vi "MicronManager.vi"() -> ()   [LabVIEW 2019]
uses:
  MicronManager.lvclass
  <vilib>/Utility/error.llb/DialogType.ctl
  <vilib>/SLL Toolkit/SLL Queued State Machine/Queue Driver/Create Queue.vi
  <vilib>/SLL Toolkit/SLL Queued State Machine/Queue Driver/Enqueue an Item to Queue.vi
  <vilib>/SLL Toolkit/SLL Queued State Machine/Queue Driver/Dequeue Queue.vi
  <vilib>/SLL Toolkit/SLL Queued State Machine/Queue Driver/Enqueue N Items.vi
  <vilib>/SLL Toolkit/SLL Easy TCP/_SubVIs/TCP Initialize Client - Local.vi
  <vilib>/SLL Toolkit/SLL String/_SubVIs/I32 to String.vi
  <vilib>/SLL Toolkit/SLL Queued State Machine/Queue Driver/Flush Queue.vi
  <vilib>/SLL Toolkit/SLL Queued State Machine/Queue Driver/Release Queue.vi
  <vilib>/SLL Toolkit/SLL Easy TCP/SLL Easy API via TCP.lvclass
  <vilib>/SLL Toolkit/SLL Queued State Machine/SLL QSM.lvlib
  <vilib>/SLL Toolkit/SLL String/SLL String.lvlib
panel:
  in  "Ping All":bool
  out "Status":string
  in  "Tab Control":enum32{"Services", "Message"}(tab)
  out "Services":string[][](table)
  in  "Service Name":string(combo)="MicronService"
  out "Read Data":string
  in  "Command":string(combo)="Ping"
  in  "Execute":bool
  in  "Service List":path=path "ServiceList.csv"
  in  "Stop All":bool
  in  "Start All":bool
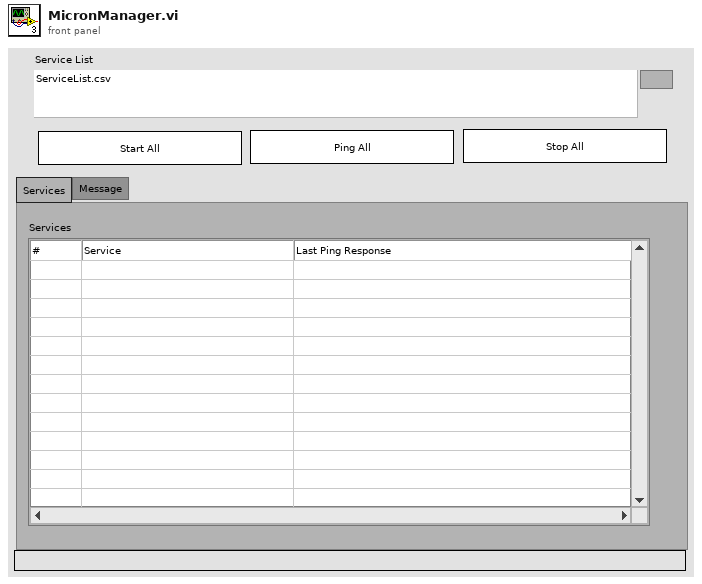
[diagram p1: front panel]
types:
  T1 = cluster{"Flags":cluster{"Source Code?":bool}, "Services":string[], "MicronManager":refnum<class "MicronManager.lvclass">, "Ping Responses":string[]}
  T2 = typedef "DialogType.ctl" = u16
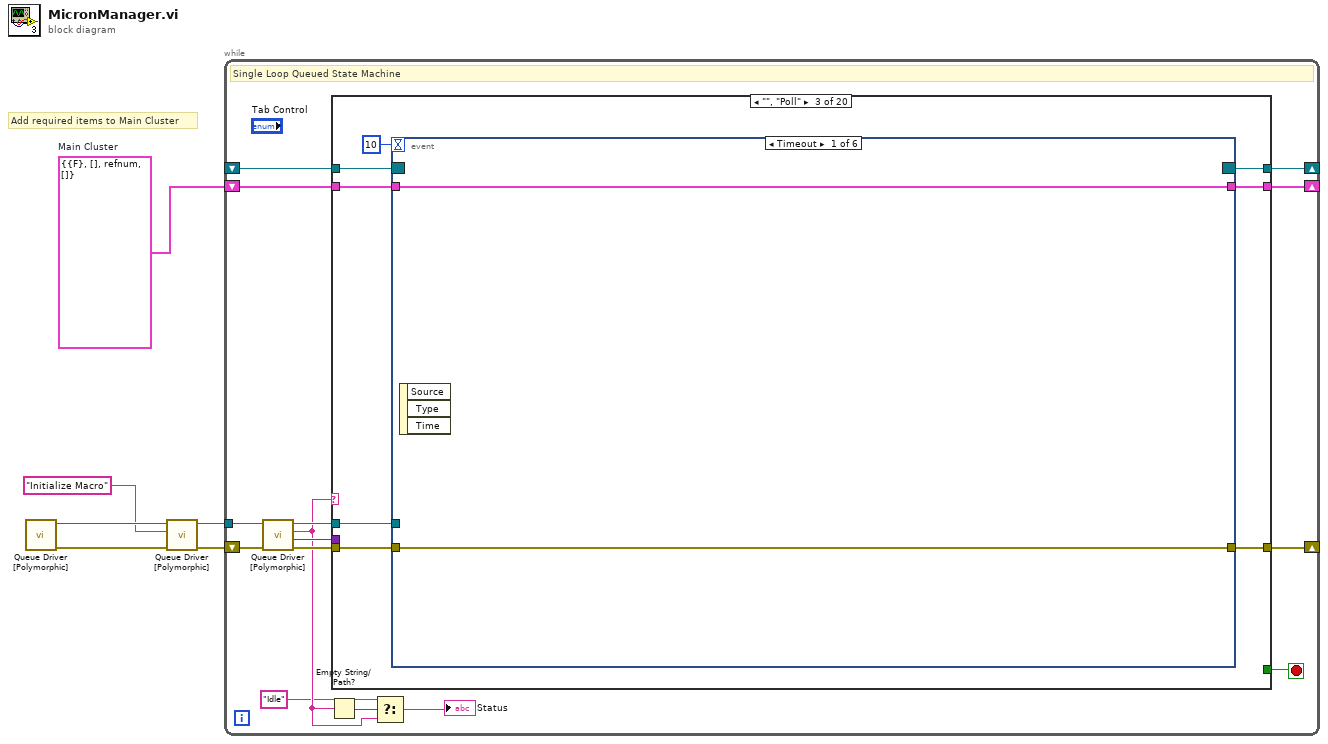
[diagram p0: block diagram]
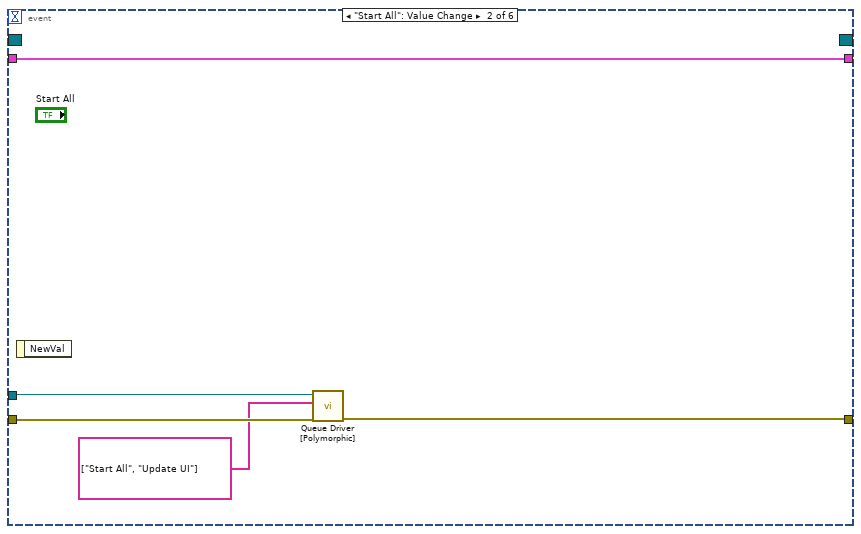
[diagram p4: hidden frame]
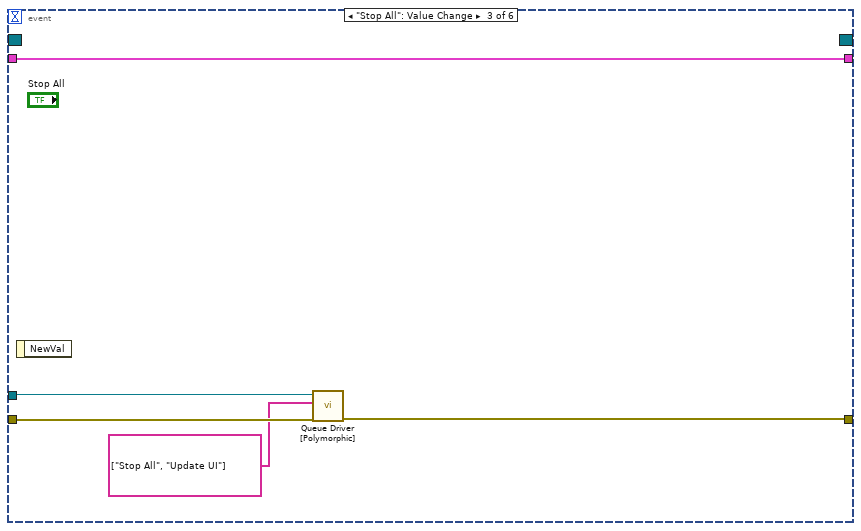
[diagram p5: hidden frame]
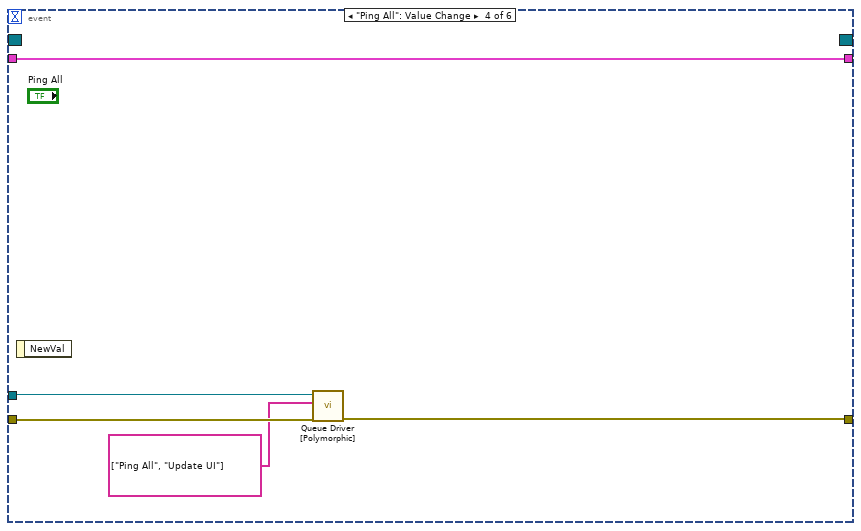
[diagram p6: hidden frame]
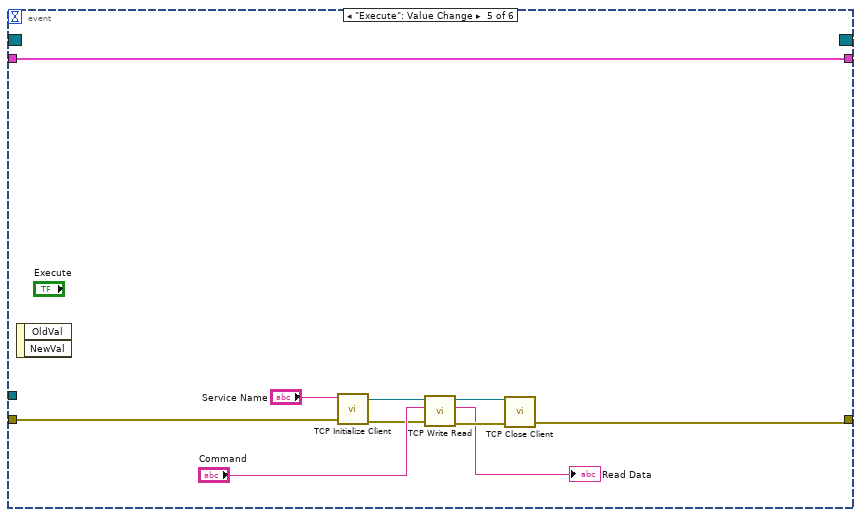
[diagram p7: hidden frame]
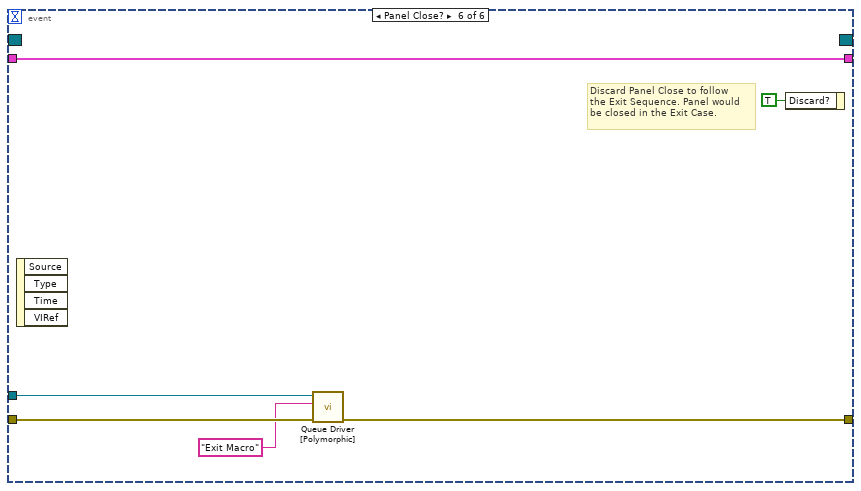
[diagram p8: hidden frame]
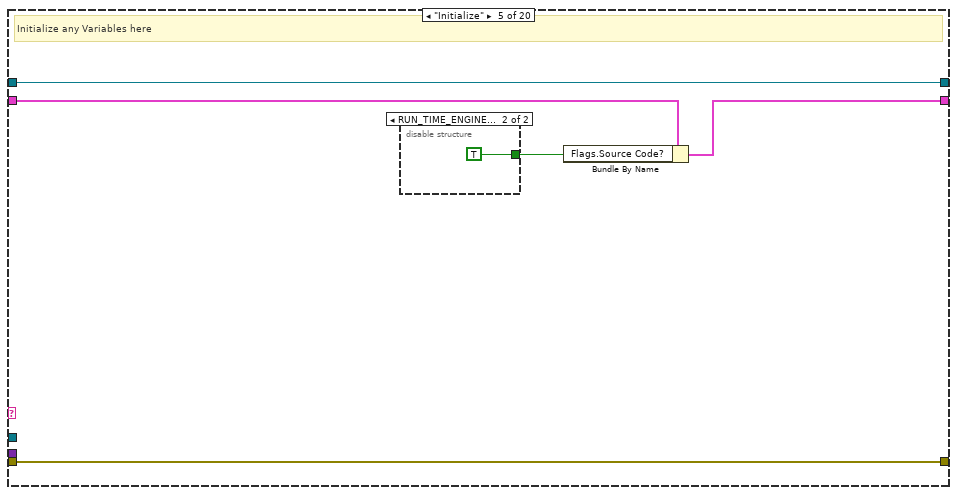
[diagram p10: hidden frame]
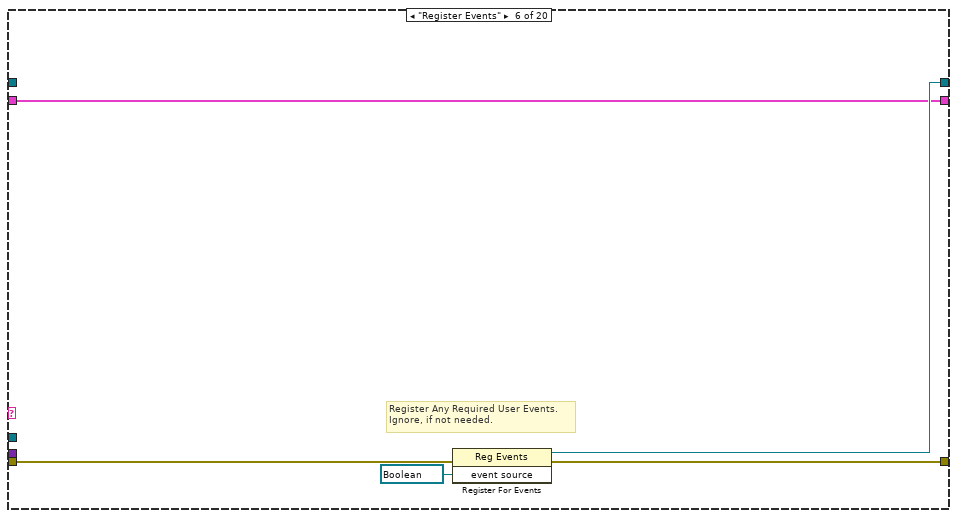
[diagram p12: hidden frame]
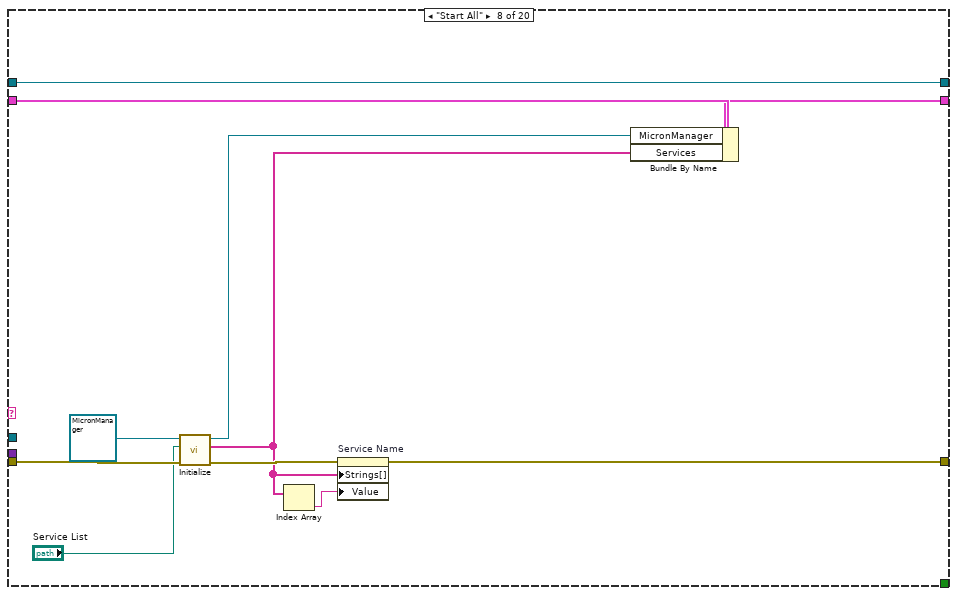
[diagram p14: hidden frame]
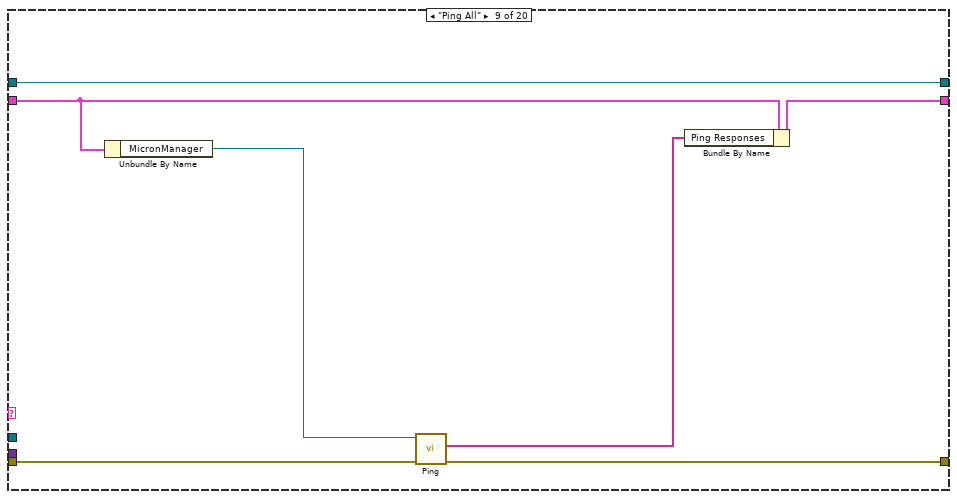
[diagram p15: hidden frame]
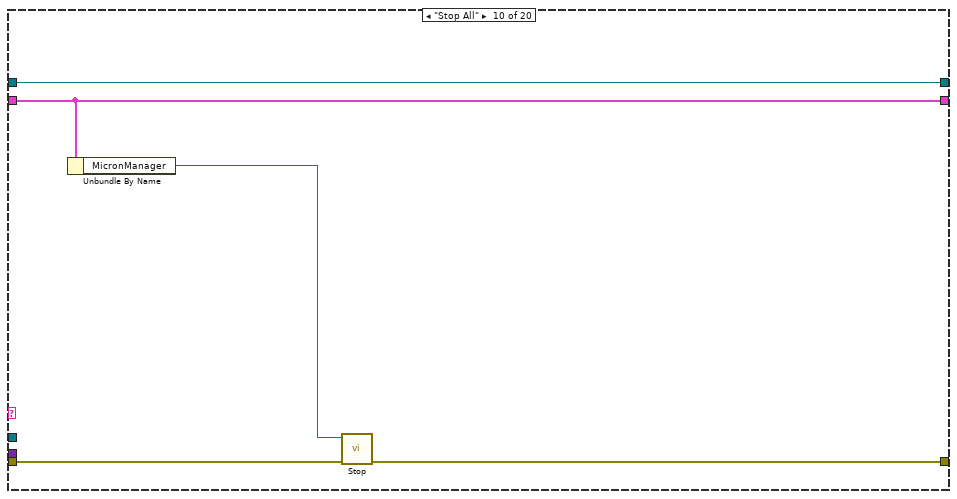
[diagram p16: hidden frame]
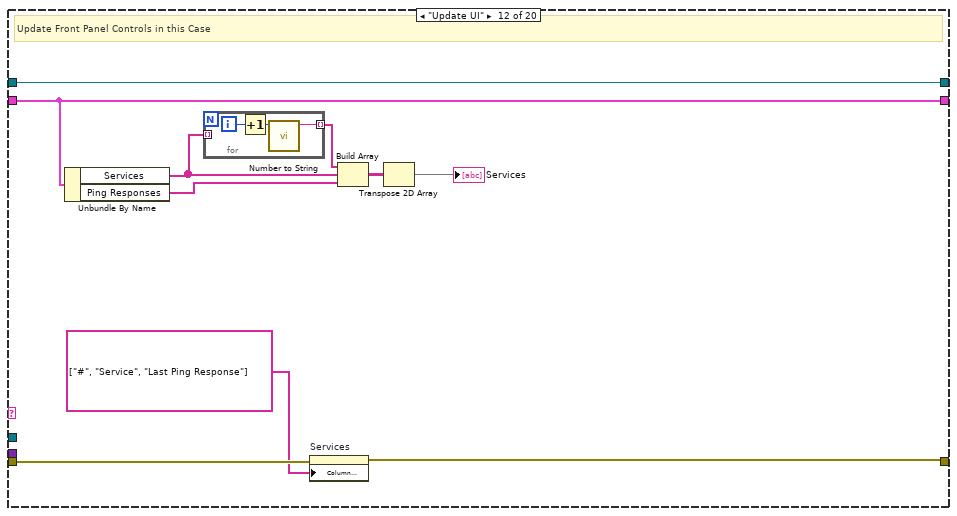
[diagram p18: hidden frame]
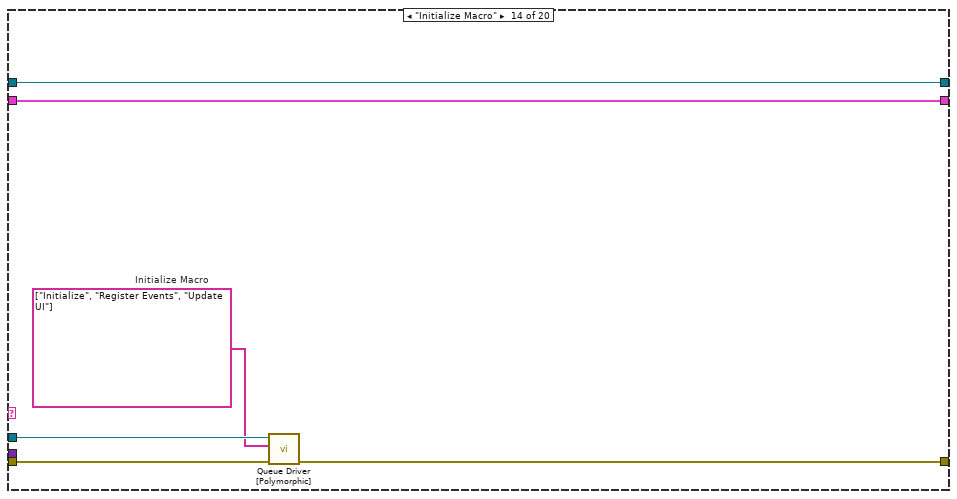
[diagram p20: hidden frame]
diagram:
  w3 = T1 {"Flags"={"Source Code?"=FALSE}, "Services"=[], "MicronManager"=refnum, "Ping Responses"=[]}  # Main Cluster
  # "Add required items to Main Cluster"
  n1 = call-poly <vilib>:"Queue Driver [Polymorphic].vi"() -> ("Error Out"=w1:errorcluster, "Queue Ref"=w5:refnum<queue>)  [unwired: 10 in]
  n2 = call-poly <vilib>:"Queue Driver [Polymorphic].vi"("Error In"=w1, "Item to Add"="Initialize Macro", "Queue Ref In"=w5) -> ("Error Out"=w2:errorcluster, "Queue Ref Out"=w6:refnum<queue>)  [unwired: 7 in]
  n3 = while "SLL Queued State Machine" {
    shift-right: [w19] -> _
    shift-left: w2 -> [w21]
    shift-right: [w17] -> _
    shift-left: _ -> [w16]
    shift-right: [w15] -> _
    shift-left: w3 -> [w14]
    tunnel: w6 -> [w13]
    stop <- w18 stop-if-true
    # "Single Loop Queued State Machine"
    n4 = call-poly <vilib>:"Queue Driver [Polymorphic].vi"("Error In"=w21, "Queue Ref In"=w13) -> ("Error Out"=w20:errorcluster, "Data"=w11:variant, "Dequeue"=w9:string, "Queue Ref Out"=w12:refnum<queue>)  [unwired: 6 in]
    n5 = Empty String/Path?(string/path=w9) -> (empty?=w10:bool)
    n6 = case "QSM Case Structure" shown="\"\", \"Poll\"" w9 {
      selector: w9 -> [_ _ _ _ _ _ _ _ _ _ _ _ _ _ _ _ w143 _ _ _]
      tunnel: w20 -> [w24 w27 w33 w71 w76 w82 w85 w92 w103 w106 w111 w117 w127 w131 w137 w142 w146 w158 w161 w178]
      tunnel: [w24 w27 w34 w71 w76 w81 w85 w95 w101 w105 w111 w116 w127 w130 w136 w142 w149 w156 w161 w164] -> w19
      tunnel: [_ _ _ _ _ _ _ _ _ _ _ _ _ _ _ _ _ _ _ TRUE] -> w18
      tunnel: [w23 w26 w32 w70 w75 w80 w84 w96 w102 w108 w110 w121 w126 w133 w139 w141 w152 w155 w160 w177] -> w17
      tunnel: w16 -> [w23 w26 w31 w70 w75 _ w84 w96 w102 w108 w110 w121 w126 w133 w139 w141 w152 w155 w160 w177]
      tunnel: [w22 w25 w29 w69 w72 w79 w83 w93 w98 w107 w109 w120 w125 w132 w138 w140 w151 w154 w159 w176] -> w15
      tunnel: w14 -> [w22 w25 w30 w69 w73 w79 w83 w94 w100 w107 w109 w120 w125 w132 w138 w140 w151 w154 w159 w176]
      tunnel: w12 -> [_ _ w28 _ _ _ _ _ _ _ _ _ _ w129 w134 _ _ _ _ w167]
      tunnel: w11 -> [_ _ _ _ _ _ _ _ _ _ _ _ _ _ _ _ _ _ _ _]
      frame "/--------------- Read Me -----------------/" {
        # "General Purpose Queue Based State Machine for Any Use Case (main application, module, pop up message etc)\n\nAdvantages:\n1. Lean Project Code Base (dependencies are in vilib).\n2. This template can be safely used in multiple parallel running modules without any issues.\n3. This template can also be safely used even in cases where the VI is configured to be a clone, where multiple \ninstances of the VI could be executing concurrently.\n\nHow to Use:\n1. Add necessary items to the Main Cluster.\n2. Use the Polymorphic Queue Driver for doing any queue operations. \n3. Add any required user events in the \"Register Events\" case. Ignore if not needed.\n4. Use \"Macros\" section for defining any list of state calls, which could be used in multiple places. \nEx: Initialize Macro, might be needed if we need to any reinitialization."
      }
      frame "/------------------ Poll -------------------/" {
      }
      frame "", "Poll" {
        n7 = event shown="[0] Timeout" {
          selector: w31 -> [_ _ _ _ _ _]
          dyn-events: [_ _ _ _ _ _] -> w32
          timeout: 10 -> [_ _ _ _ _ _]
          tunnel: [w37 w40 w45 w50 w53 w67] -> w34
          tunnel: w33 -> [w37 w41 w46 w51 w54 w68]
          tunnel: w30 -> [w36 w42 w47 w52 w62 w66]
          tunnel: [w36 w42 w47 w52 w62 w66] -> w29
          tunnel: w28 -> [_ w39 w44 w49 _ w64]
          event Timeout {
            n8 = event-data() -> ()  [unwired: 1 in, 3 out]
          }
          event "Start All": Value Change {
            n9 = event-data() -> ()  [unwired: 1 in, 1 out]
            n10 = call-poly <vilib>:"Queue Driver [Polymorphic].vi"("Error In"=w41, "Enqueue N"=string[] ["Start All", "Update UI"], "Queue Ref In"=w39) -> ("Error Out"=w40:errorcluster)  [unwired: 7 in, 1 out]
          }
          event "Stop All": Value Change {
            n11 = event-data() -> ()  [unwired: 1 in, 1 out]
            n12 = call-poly <vilib>:"Queue Driver [Polymorphic].vi"("Error In"=w46, "Enqueue N"=string[] ["Stop All", "Update UI"], "Queue Ref In"=w44) -> ("Error Out"=w45:errorcluster)  [unwired: 7 in, 1 out]
          }
          event "Ping All": Value Change {
            n13 = event-data() -> ()  [unwired: 1 in, 1 out]
            n14 = call-poly <vilib>:"Queue Driver [Polymorphic].vi"("Error In"=w51, "Enqueue N"=string[] ["Ping All", "Update UI"], "Queue Ref In"=w49) -> ("Error Out"=w50:errorcluster)  [unwired: 7 in, 1 out]
          }
          event "Execute": Value Change {
            n15 = event-data() -> ()  [unwired: 1 in, 2 out]
            n16 = call-poly <vilib>:"TCP Initialize Client.vi"("error in (no error)"=w54, "Service Name"="Service Name") -> ("error out"=w58:errorcluster, "connection ID Out"=w55:refnum<k5>)  [unwired: 8 in]
            n17 = call <vilib>:"TCP Write Read.vi"("error in (no error)"=w58, "Write Data"="Command", "connection ID In"=w55) -> ("error out"=w59:errorcluster, "Read Data"=→"Read Data":string, "connection ID Out"=w56:refnum<k5>)  [unwired: 5 in, 1 out]
            n18 = call <vilib>:"TCP Close Client.vi"("error in (no error)"=w59, "connection ID"=w56) -> ("error out"=w53:errorcluster)  [unwired: 9 in]
          }
          event Panel Close? {
            # "Discard Panel Close to follow\nthe Exit Sequence. Panel would\nbe closed in the Exit Case."
            n19 = event-data() -> ()  [unwired: 1 in, 4 out]
            n20 = call-poly <vilib>:"Queue Driver [Polymorphic].vi"("Error In"=w68, "Item to Add"="Exit Macro" ("Enqueue"), "Queue Ref In"=w64) -> ("Error Out"=w67:errorcluster)  [unwired: 7 in, 1 out]
            n21 = event-data("Discard?"=TRUE) -> ()  [unwired: 1 in, 1 out]
          }
        }
      }
      frame "/--------------- Initialize -----------------/" {
      }
      frame "Initialize" {
        # "Initialize any Variables here"
        n22 = disable-structure shown="RUN_TIME_ENGINE==False" {
          disable-tunnel: [_ TRUE] -> w74
          frame condition #0 {
          }
          frame condition #1 (active) {
          }
        }
        n23 = Bundle By Name(cluster=w73, "Flags.Source Code?"=w74) -> (w72:T1)
      }
      frame "Register Events" {
        # "Register Any Required User Events. \nIgnore, if not needed."
        n24 = register-events(error in=w82, refnum<vi> refnum ("event source")) -> (reference out=w80:refnum<event-registration>, error out=w81:errorcluster)  [unwired: 1 in]
      }
      frame "/---------- Custom Case Splitter ----------/" {
      }
      frame "Start All" {
        n25 = call-dynamic "Initialize.vi"("error in (no error)"=w92, "Service List"="Service List", "MicronManager in"=refnum<class "MicronManager.lvclass"> refnum) -> ("error out"=w91:errorcluster, "Services"=w87:string[], "MicronManager out"=w89:refnum<class "MicronManager.lvclass">)  [unwired: 6 in]
        n26 = Index Array(array=w87) -> (element=w86:string)  [unwired: 1 in]
        n27 = property on="Service Name" class="CmbBox"(error in=w91, "Strings[]"=w87, "Value"=w86) -> (error out=w95:errorcluster)  [unwired: 1 in, 1 out]
        n28 = Bundle By Name(cluster=w94, "MicronManager"=w89, "Services"=w87) -> (w93:T1)
      }
      frame "Ping All" {
        n29 = Unbundle By Name(w100) -> ("MicronManager"=w99:refnum<class "MicronManager.lvclass">)
        n30 = call-dynamic "Ping.vi"("error in (no error)"=w103, "MicronManager in"=w99) -> ("error out"=w101:errorcluster, "Responses"=w97:string[])  [unwired: 7 in, 1 out]
        n31 = Bundle By Name(cluster=w100, "Ping Responses"=w97) -> (w98:T1)
      }
      frame "Stop All" {
        n32 = Unbundle By Name(w107) -> ("MicronManager"=w104:refnum<class "MicronManager.lvclass">)
        n33 = call-dynamic "Stop.vi"("error in (no error)"=w106, "MicronManager in"=w104) -> ("error out"=w105:errorcluster)  [unwired: 8 in, 1 out]
      }
      frame "/-------------- User Interface --------------/" {
        # "Duplicate this case to create additional case splitters for readability"
      }
      frame "Update UI" {
        # "Update Front Panel Controls in this Case"
        n34 = Unbundle By Name(w120) -> ("Services"=w114:string[], "Ping Responses"=w119:string[])
        n35 = for {
          tunnel: w114 -> [_] mode=indexing
          tunnel: [w123] -> w113 mode=indexing
          i -> [w124]
          n36 = Increment(x=w124) -> (x+1=w122:i32)
          n37 = call-poly <vilib>:"Number to String.vi"("Numeric"=w122) -> ("String"=w123:string)  [unwired: 10 in]
        }
        n38 = property on="Services" class="Tbl (strict)"(error in=w117, "Column Headers[]"=string[] ["#", "Service", "Last Ping Response"]) -> (error out=w116:errorcluster)  [unwired: 1 in, 1 out]
        n39 = Build Array(w113, w114, w119) -> (w118:string[][])
        n40 = Transpose 2D Array(2D array=w118) -> (transposed array=→"Services":string[][])
      }
      frame "/----------------- Macros -----------------/" {
      }
      frame "Initialize Macro" {
        w128 = string[] ["Initialize", "Register Events", "Update UI"]  # Initialize Macro
        n41 = call-poly <vilib>:"Queue Driver [Polymorphic].vi"("Error In"=w131, "Enqueue N"=w128, "Queue Ref In"=w129) -> ("Error Out"=w130:errorcluster)  [unwired: 7 in, 1 out]
      }
      frame "Exit Macro" {
        n42 = call-poly <vilib>:"Queue Driver [Polymorphic].vi"("Error In"=w137, "Enqueue N"=string[] ["Exit"], "Queue Ref In"=w134) -> ("Error Out"=w136:errorcluster)  [unwired: 7 in, 1 out]
      }
      frame "/-------------- Error Handler--------------/" {
      }
      frame Default {
        # "Undefined Case/Spelling Errors - Show Message to Developer"
        n43 = property class="VI"(error in=w146) -> (error out=w145:errorcluster, "Name"=w144:string)  [unwired: 1 in, 1 out]
        n44 = Format Into String(format string="\"%s\" in the VI - %s" ("message"), initial string="Undefined case - ", error in=w145, w143, w144) -> (resulting string=w147:string, error out=w149:errorcluster)
        n45 = One Button Dialog(message=w147) -> ()  [unwired: 1 in, 1 out]
      }
      frame "Error" {
        w153 = T2 2 items=["no dialog", "OK message", "continue or stop message", "OK message + warnings", "continue/stop + warnings"] ("type of dialog (OK msg:1)")
        # "Handle the Error"
        n46 = call <vilib>:"Simple Error Handler.vi"("type of dialog (OK msg:1)"=w153, "error in (no error)"=w158) -> ("error out"=w157:errorcluster)  [unwired: 3 in, 4 out]
        n47 = call <vilib>:"Clear Errors.vi"("error in (no error)"=w157) -> ("error out"=w156:errorcluster)  [unwired: 5 in, 1 out]
      }
      frame "/------------------- Exit --------------------/" {
      }
      frame "Exit" {
        n48 = call-poly <vilib>:"Queue Driver [Polymorphic].vi"("Error In"=w178, "Queue Ref In"=w167) -> ("Error Out"=w179:errorcluster, "Queue Ref Out"=w166:refnum<queue>)  [unwired: 7 in, 1 out]
        n49 = Unbundle By Name(w176) -> ("Flags.Source Code?"=w169:bool)
        n50 = call-poly <vilib>:"Queue Driver [Polymorphic].vi"("Error In"=w179, "Queue Ref In"=w166) -> ("Error Out"=w175:errorcluster)  [unwired: 9 in]
        n51 = Call Chain() -> (call chain=w173:string[])
        n52 = Array Size(array=w173) -> (size(s)=w172:i32)
        n53 = Equal?(x=w172, y=1) -> (x = y?=w170:bool)
        n54 = And(x=w169, y=w170) -> (x .and. y?=w168:bool)
        n55 = case "Skip Panel Close when in Source\nCode and is the top most caller" shown="False" w168 {
          tunnel: w175 -> [w182 w184]
          tunnel: [w183 w184] -> w174
          frame False {
            # "Close Panel"
            n56 = invoke class="VI" method="FP.Close"() -> (error out=w181:errorcluster)  [unwired: 3 in, 2 out]
            n57 = Merge Errors(w182, w181) -> (w183:errorcluster)
          }
          frame True {
            # "Do Not Close Panel"
          }
        }
        n58 = invoke class="VI" method="Default Vals.Reinit All"(error in=w174) -> (error out=w165:errorcluster)  [unwired: 2 in, 2 out]
        n59 = property on="Service Name" class="CmbBox"(error in=w165, "Strings[]"=string[] [] ("Strings []"), "Value"="") -> (error out=w164:errorcluster)  [unwired: 1 in, 1 out]
      }
    }
    n60 = Select(t="Idle", s=w10, f=w9) -> (s? t:f=→"Status":string)
  }
